vi "case_start_torture.vi"(5 "Uninitialized message":string, 7 "initialized":bool, 8 "error in (no error)":errorcluster, 9 "Main VI reference":refnum<vi>, 10 "queue in":refnum<queue>, 11 "VISA Refnum in":refnum<visa-resource-name>) -> (0 "error out":errorcluster, 3 "VISA Refnum out":refnum<visa-resource-name>)   [LabVIEW 2020]
uses:
  controls/message cluster.ctl
  <instrlib>/Marlin Instrument Driver/Public/controls/move parameters.ctl
  05ddde7c-8748-41b3-8414-943d1f29c513.vi
  d9742ba0-ac86-45fc-b336-184dcbcfad4f.vi
  f3d951a2-545d-464d-8711-b5a225ef32bc.vi
  850a9ad7-1773-40e0-ba22-3ffedd80f675.vi
  8aa21fe5-c641-49fc-ade5-270ce292e105.vi
  31cc3a57-414c-49b1-b22e-c1078cf77971.vi
  <instrlib>/Marlin Instrument Driver/Marlin Instrument Driver.lvlib
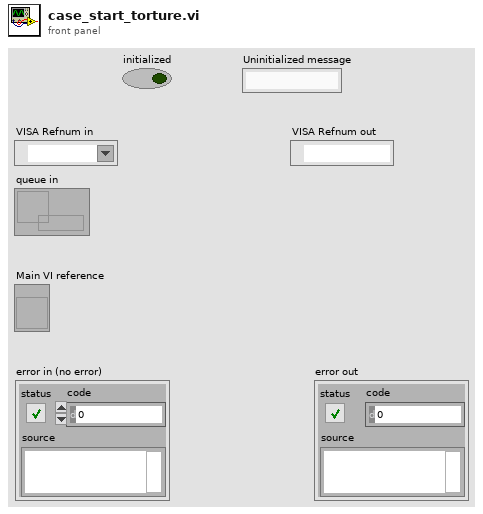
[diagram p1: front panel]
types:
  T1 = typedef "message cluster.ctl" = cluster{"message":string, "data":variant}
  T2 = typedef "Marlin Instrument Driver.lvlib/move parameters.ctl" = cluster{"E":dbl, "F":dbl, "X":dbl, "Y":dbl, "Z":dbl}
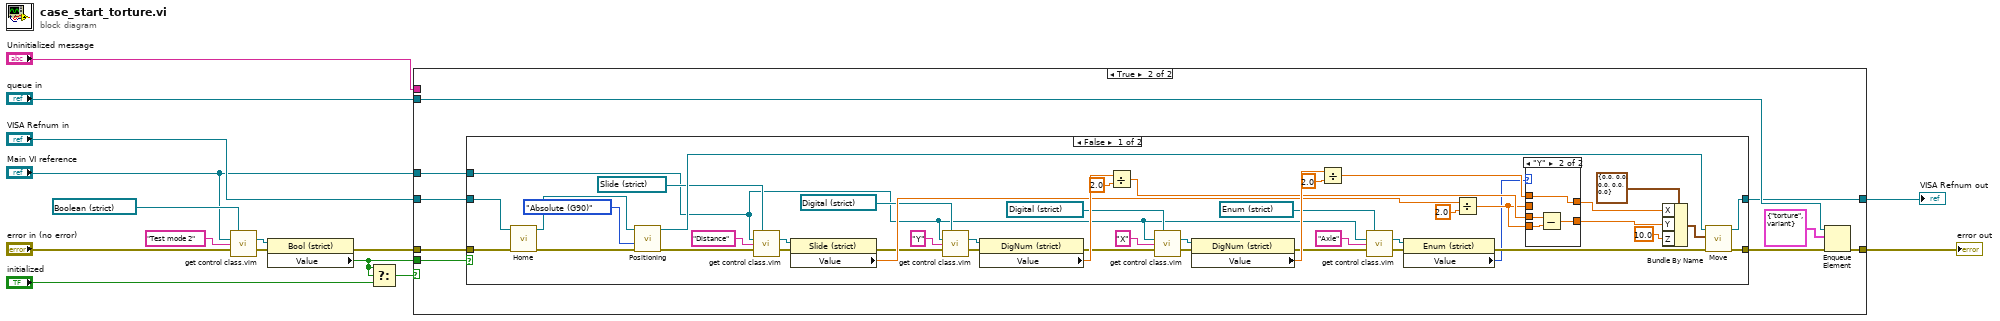
[diagram p0: block diagram]
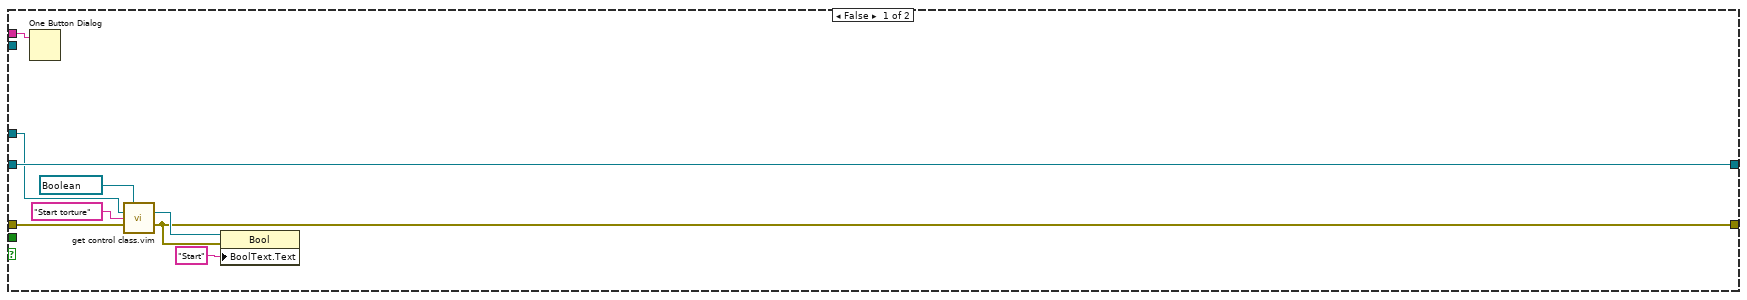
[diagram p2: hidden frame]
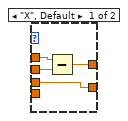
[diagram p3: hidden frame]
diagram:
  n1 = call "get control class.vim"("Control class"=refnum<vi> refnum ("Test mode 2"), "Main VI reference"="Main VI reference", "Label"="Test mode 2", "error in (no error)"="error in (no error)") -> ("Control out"=w6:refnum<vi>, "error out"=w5:errorcluster)  [unwired: 10 in]
  n2 = property class="Bool (strict)"(reference=w6, error in=w5) -> (error out=w1:errorcluster, "Value"=w4:bool)  [unwired: 1 out]
  n3 = Select(t=w4, s=w4, f="initialized") -> (s? t:f=w13:bool)
  n4 = case shown="True" w13 {
    tunnel: "VISA Refnum in" -> [w24 w33]
    tunnel: w1 -> [w18 w32]
    tunnel: "queue in" -> [_ w31]
    tunnel: [w17 w29] -> w11
    tunnel: [w24 w27] -> w12
    tunnel: "Uninitialized message" -> [w23 _]
    tunnel: w4 -> [_ w26]
    tunnel: "Main VI reference" -> [w16 w25]
    frame False {
      n5 = One Button Dialog(message=w23) -> ()  [unwired: 1 in, 1 out]
      n6 = call "get control class.vim"("Control class"=refnum<vi> refnum ("Start torture"), "Main VI reference"=w16, "Label"="Start torture", "error in (no error)"=w18) -> ("Control out"=w19:refnum<vi>, "error out"=w17:errorcluster)  [unwired: 10 in]
      n7 = property on="Property Node" class="Bool"(reference=w19, error in=w17, "BoolText.Text"="Start" ("Boolean Text.Text")) -> ()  [unwired: 2 out]
    }
    frame True {
      n8 = case shown="False" w26 {
        tunnel: w33 -> [w67 w87]
        tunnel: w32 -> [w53 w88]
        tunnel: [w59 w88] -> w28
        tunnel: [w58 w87] -> w27
        tunnel: w25 -> [w34 _]
        frame False {
          n9 = call <instrlib>:"Home.vi"("error in (no error)"=w53, "VISA resource name"=w67) -> ("error out"=w69:errorcluster, "VISA resource name out"=w68:refnum<visa-resource-name>)  [unwired: 8 in]
          n10 = call <instrlib>:"Positioning.vi"("error in (no error)"=w69, "type"=enum16{"Absolute (G90)", "Relative (G91)"}."Absolute (G90)", "VISA resource name"=w68) -> ("error out"=w52:errorcluster, "VISA resource name out"=w78:refnum<visa-resource-name>)  [unwired: 7 in]
          n11 = call "get control class.vim"("Control class"=refnum<vi> refnum ("Distance"), "Main VI reference"=w34, "Label"="Distance", "error in (no error)"=w52) -> ("Control out"=w54:refnum<vi>, "error out"=w55:errorcluster)  [unwired: 10 in]
          n12 = property on="Property Node" class="Slide (strict)"(reference=w54, error in=w55) -> (error out=w47:errorcluster, "Value"=w65:dbl)  [unwired: 1 out]
          n13 = call "get control class.vim"("Control class"=refnum<vi> refnum ("X"), "Main VI reference"=w34, "Label"="Y", "error in (no error)"=w47) -> ("Control out"=w49:refnum<vi>, "error out"=w48:errorcluster)  [unwired: 10 in]
          n14 = property on="Property Node" class="DigNum (strict)"(reference=w49, error in=w48) -> (error out=w42:errorcluster, "Value"=w73:dbl)  [unwired: 1 out]
          n15 = Divide(x=w73, y=2.0) -> (x/y=w61:dbl)
          n16 = call "get control class.vim"("Control class"=refnum<vi> refnum ("X"), "Main VI reference"=w34, "Label"="X", "error in (no error)"=w42) -> ("Control out"=w43:refnum<vi>, "error out"=w44:errorcluster)  [unwired: 10 in]
          n17 = property on="Property Node" class="DigNum (strict)"(reference=w43, error in=w44) -> (error out=w37:errorcluster, "Value"=w76:dbl)  [unwired: 1 out]
          n18 = Divide(x=w76, y=2.0) -> (x/y=w63:dbl)
          n19 = call "get control class.vim"("Control class"=refnum<vi> refnum ("Axle"), "Main VI reference"=w34, "Label"="Axle", "error in (no error)"=w37) -> ("Control out"=w40:refnum<vi>, "error out"=w41:errorcluster)  [unwired: 10 in]
          n20 = property class="Enum (strict)"(reference=w40, error in=w41) -> (error out=w36:errorcluster, "Value"=w35:enum16{"X", "Y", "Z"})  [unwired: 1 out]
          n21 = Divide(x=w65, y=2.0) -> (x/y=w60:dbl)
          n22 = case shown="\"Y\"" w35 {
            tunnel: [w80 w86] -> w64
            tunnel: w63 -> [w81 w86]
            tunnel: w60 -> [w82 _]
            tunnel: [w79 w83] -> w62
            tunnel: w61 -> [w79 w84]
            tunnel: w60 -> [_ w85]
            frame "X", Default {
              n23 = Subtract(x=w81, y=w82) -> (x-y=w80:dbl)
            }
            frame "Y" {
              n24 = Subtract(x=w84, y=w85) -> (x-y=w83:dbl)
            }
          }
          n25 = Bundle By Name(cluster=T2 {"E"=0.0, "F"=0.0, "X"=0.0, "Y"=0.0, "Z"=0.0} ("Distances"), "X"=w64, "Y"=w62, "Z"=10.0) -> (w70:T2)
          n26 = call <instrlib>:"Move.vi"("error in (no error)"=w36, "Distances"=w70, "VISA resource name"=w78) -> ("error out"=w59:errorcluster, "VISA resource name out"=w58:refnum<visa-resource-name>)  [unwired: 7 in]
        }
        frame True {
        }
      }
      n27 = Enqueue Element(queue=w31, element=T1 {"message"="torture", "data"=variant}, error in (no error)=w28) -> (error out=w29:errorcluster)  [unwired: 1 in, 2 out]
    }
  }
  "VISA Refnum out" <- w12
  "error out" <- w11
